vi "USB3 Convert Driver Err To Windows Err.vi"(8 "error in (no error)":errorcluster, 9 "peDriverErrorType":u32(ring) items=["eDriverInvalidError", "eDriverNtStatus", "eDriverUsbdStatus"], 10 "pnWindowsErrorCode":i32, 11 "nErrorCode":i32) -> (0 "error out":errorcluster, 1 "peDriverErrorType out":u32(ring) items=["eDriverInvalidError", "eDriverNtStatus", "eDriverUsbdStatus"], 2 "pnWindowsErrorCode out":i32, 3 "function return":i32)   [LabVIEW 2013, in "Octoplus_LIDAR.lvlib"]
doc: "CAMCMOSOCTUSB3_API int __cdecl USB3_ConvertDriverErrToWindowsErr(int nErrorCode, int * pnWindowsErrorCode, tDriverErrorType * peDriverErrorType);"
uses:
  <userlib>/Octoplus_LIDAR/Octoplus_LIDAR.lvlib
  <userlib>/Octoplus_LIDAR/CamCmosOctUsb3.dll
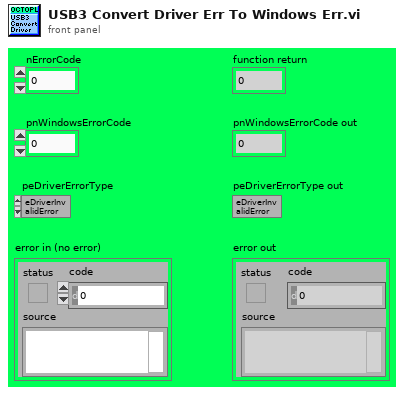
[diagram p1: front panel]
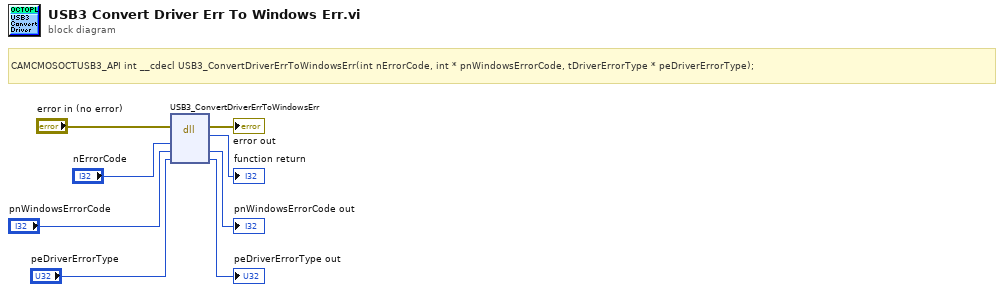
[diagram p0: block diagram]
diagram:
  # "CAMCMOSOCTUSB3_API int __cdecl USB3_ConvertDriverErrToWindowsErr(int nErrorCode, int * pnWindowsErrorCode, tDriverErrorType * peDriverErrorType);"
  n1 = dll-call lib="C:/Program Files/National Instruments/LabVIEW 2013/user.lib/Octoplus_LIDAR/CamCmosOctUsb3.*" fn="USB3_ConvertDriverErrToWindowsErr"(error in="error in (no error)", "nErrorCode"="nErrorCode", "pnWindowsErrorCode"="pnWindowsErrorCode", "peDriverErrorType"="peDriverErrorType") -> (error out=→"error out":errorcluster, →"function return":i32, "pnWindowsErrorCode"=→"pnWindowsErrorCode out":i32, "peDriverErrorType"=→"peDriverErrorType out":u32)  [unwired: 3 in, 1 out]
